vi "Settling Delay Control.vi"(7 "error in":errorcluster, 8 "Settings Cluster":T1={"Supply Voltage [Vdc]"=0.0, "Max Supply Current [Idc]"=0.0, "Settling Delay"=0.0, "Temp Criteria"=0.0, "Voltage Steps [Vrms]"=[], "User Notes"="", "Config Wave File Path"=path "", "Config Voltage [Vrms]"=0.0, "Channel Configuration List"={"Channel Configuration Cluster"={"Input"=enum."---", "Enable"=FALSE, "User Notes"="", "Voltage Range"=15.0, "Current Range"=2.5}, "Channel Configuration Cluster 2"={"Input"=enum."---", "Enable"=FALSE, "User Notes"="", "Voltage Range"=15.0, "Current Range"=2.5}, "Channel Configuration Cluster 3"={"Input"=enum."---", "Enable"=FALSE, "User Notes"="", "Voltage Range"=15.0, "Current Range"=2.5}, "Channel Configuration Cluster 4"={"Input"=enum."---", "Enable"=FALSE, "User Notes"="", "Voltage Range"=15.0, "Current Range"=2.5}, "Channel Configuration Cluster 5"={"Input"=enum."---", "Enable"=FALSE, "User Notes"="", "Voltage Range"=15.0, "Current Range"=2.5}, "Channel Configuration Cluster 6"={"Input"=enum."---", "Enable"=FALSE, "User Notes"="", "Voltage Range"=15.0, "Current Range"=2.5}, "Channel Configuration Cluster 7"={"Input"=enum."---", "Enable"=FALSE, "User Notes"="", "Voltage Range"=15.0, "Current Range"=2.5}, "Channel Configuration Cluster 8"={"Input"=enum."---", "Enable"=FALSE, "User Notes"="", "Voltage Range"=15.0, "Current Range"=2.5}, "Channel Configuration Cluster 9"={"Input"=enum."---", "Enable"=FALSE, "User Notes"="", "Voltage Range"=15.0, "Current Range"=2.5}, "Channel Configuration Cluster 10"={"Input"=enum."---", "Enable"=FALSE, "User Notes"="", "Voltage Range"=15.0, "Current Range"=25.0}, "Channel Configuration Cluster 11"={"Input"=enum."---", "Enable"=FALSE, "User Notes"="", "Voltage Range"=15.0, "Current Range"=25.0}, "Channel Configuration Cluster 12"={"Input"=enum."---", "Enable"=FALSE, "User Notes"="", "Voltage Range"=15.0, "Current Range"=25.0}, "Channel Configuration Cluster 13"={"Input"=enum."---", "Enable"=FALSE, "User Notes"="", "Voltage Range"=15.0, "Current Range"=25.0}, "Channel Configuration Cluster 14"={"Input"=enum."---", "Enable"=FALSE, "User Notes"="", "Voltage Range"=15.0, "Current Range"=25.0}, "Channel Configuration Cluster 15"={"Input"=enum."---", "Enable"=FALSE, "User Notes"="", "Voltage Range"=15.0, "Current Range"=25.0}, "Channel Configuration Cluster 16"={"Input"=enum."---", "Enable"=FALSE, "User Notes"="", "Voltage Range"=15.0, "Current Range"=25.0}, "Channel Configuration Cluster 17"={"Input"=enum."---", "Enable"=FALSE, "User Notes"="", "Voltage Range"=15.0, "Current Range"=25.0}}, "User Gains"={"Gain 1"=0.0, "Gain 2"=0.0, "Gain 3"=0.0, "Gain 4"=0.0, "Gain 5"=0.0, "Gain 6"=0.0}, "Gains"={"Gain 1"=0.0, "Gain 2"=0.0, "Gain 3"=0.0, "Gain 4"=0.0, "Gain 5"=0.0, "Gain 6"=0.0}, "Gain Array"={"Gain 1"=0.0, "Gain 2"=0.0, "Gain 3"=0.0, "Gain 4"=0.0, "Gain 5"=0.0, "Gain 6"=0.0, "Gain 7"=0.0, "Gain 8"=0.0, "Gain 9"=0.0, "Gain 10"=0.0, "Gain 11"=0.0, "Gain 12"=0.0, "Gain 13"=0.0, "Gain 14"=0.0, "Gain 15"=0.0, "Gain 16"=0.0, "Gain 17"=0.0}, "Wave File Path 1"=path "", "Wave File Path 2"=path "", "Wave File Path 3"=path "", "Wave File Path 4"=path "", "Range"=FALSE, "CF"=FALSE} {"Gain Array"."Gain 17" format="%.2f"; "Gain Array"."Gain 16" format="%.2f"; "Gain Array"."Gain 15" format="%.2f"; "Gain Array"."Gain 14" format="%.2f"; "Gain Array"."Gain 13" format="%.2f"; "Gain Array"."Gain 12" format="%.2f"; "Gain Array"."Gain 11" format="%.2f"; "Gain Array"."Gain 10" format="%.2f"; "Gain Array"."Gain 9" format="%.2f"; "Gain Array"."Gain 8" format="%.2f"; "Gain Array"."Gain 7" format="%.2f"; "Gain Array"."Gain 6" format="%.2f"; "Gain Array"."Gain 5" format="%.2f"; "Gain Array"."Gain 4" format="%.2f"; "Gain Array"."Gain 3" format="%.2f"; "Gain Array"."Gain 2" format="%.2f"; "Gain Array"."Gain 1" format="%.2f"; "Gains"."Gain 6" format="%.2f"; "Gains"."Gain 5" format="%.2f"; "Gains"."Gain 4" format="%.2f"; "Gains"."Gain 3" format="%.2f"; "Gains"."Gain 2" format="%.2f"; "Gains"."Gain 1" format="%.2f"; "User Gains"."Gain 6" format="%.2f"; "User Gains"."Gain 5" format="%.2f"; "User Gains"."Gain 4" format="%.2f"; "User Gains"."Gain 3" format="%.2f"; "User Gains"."Gain 2" format="%.2f"; "User Gains"."Gain 1" format="%.2f"; "Channel Configuration List"."Channel Configuration Cluster 17"."Current Range" items=["1 <500m>"=0.5, "2 <1>"=1.0, "5 <2.5>"=2.5, "10 <5>"=5.0, "20 <10>"=10.0, "50 <25>"=25.0]; "Channel Configuration List"."Channel Configuration Cluster 17"."Voltage Range" items=["1.5 <0.75>"=0.75, "3 <1.5>"=1.5, "6 <3>"=3.0, "10 <5>"=5.0, "15 <7.5>"=7.5, "30 <15>"=15.0, "60 <30>"=30.0, "100 <50>"=50.0, "150 <75>"=75.0, "300 <150>"=150.0, "600 <300>"=300.0, "1000 <500>"=500.0]; "Channel Configuration List"."Channel Configuration Cluster 16"."Current Range" items=["1 <500m>"=0.5, "2 <1>"=1.0, "5 <2.5>"=2.5, "10 <5>"=5.0, "20 <10>"=10.0, "50 <25>"=25.0]; "Channel Configuration List"."Channel Configuration Cluster 16"."Voltage Range" items=["1.5 <0.75>"=0.75, "3 <1.5>"=1.5, "6 <3>"=3.0, "10 <5>"=5.0, "15 <7.5>"=7.5, "30 <15>"=15.0, "60 <30>"=30.0, "100 <50>"=50.0, "150 <75>"=75.0, "300 <150>"=150.0, "600 <300>"=300.0, "1000 <500>"=500.0]; "Channel Configuration List"."Channel Configuration Cluster 15"."Current Range" items=["1 <500m>"=0.5, "2 <1>"=1.0, "5 <2.5>"=2.5, "10 <5>"=5.0, "20 <10>"=10.0, "50 <25>"=25.0]; "Channel Configuration List"."Channel Configuration Cluster 15"."Voltage Range" items=["1.5 <0.75>"=0.75, "3 <1.5>"=1.5, "6 <3>"=3.0, "10 <5>"=5.0, "15 <7.5>"=7.5, "30 <15>"=15.0, "60 <30>"=30.0, "100 <50>"=50.0, "150 <75>"=75.0, "300 <150>"=150.0, "600 <300>"=300.0, "1000 <500>"=500.0]; "Channel Configuration List"."Channel Configuration Cluster 14"."Current Range" items=["1 <500m>"=0.5, "2 <1>"=1.0, "5 <2.5>"=2.5, "10 <5>"=5.0, "20 <10>"=10.0, "50 <25>"=25.0]; "Channel Configuration List"."Channel Configuration Cluster 14"."Voltage Range" items=["1.5 <0.75>"=0.75, "3 <1.5>"=1.5, "6 <3>"=3.0, "10 <5>"=5.0, "15 <7.5>"=7.5, "30 <15>"=15.0, "60 <30>"=30.0, "100 <50>"=50.0, "150 <75>"=75.0, "300 <150>"=150.0, "600 <300>"=300.0, "1000 <500>"=500.0]; "Channel Configuration List"."Channel Configuration Cluster 13"."Current Range" items=["1 <500m>"=0.5, "2 <1>"=1.0, "5 <2.5>"=2.5, "10 <5>"=5.0, "20 <10>"=10.0, "50 <25>"=25.0]; "Channel Configuration List"."Channel Configuration Cluster 13"."Voltage Range" items=["1.5 <0.75>"=0.75, "3 <1.5>"=1.5, "6 <3>"=3.0, "10 <5>"=5.0, "15 <7.5>"=7.5, "30 <15>"=15.0, "60 <30>"=30.0, "100 <50>"=50.0, "150 <75>"=75.0, "300 <150>"=150.0, "600 <300>"=300.0, "1000 <500>"=500.0]; "Channel Configuration List"."Channel Configuration Cluster 12"."Current Range" items=["1 <500m>"=0.5, "2 <1>"=1.0, "5 <2.5>"=2.5, "10 <5>"=5.0, "20 <10>"=10.0, "50 <25>"=25.0]; "Channel Configuration List"."Channel Configuration Cluster 12"."Voltage Range" items=["1.5 <0.75>"=0.75, "3 <1.5>"=1.5, "6 <3>"=3.0, "10 <5>"=5.0, "15 <7.5>"=7.5, "30 <15>"=15.0, "60 <30>"=30.0, "100 <50>"=50.0, "150 <75>"=75.0, "300 <150>"=150.0, "600 <300>"=300.0, "1000 <500>"=500.0]; "Channel Configuration List"."Channel Configuration Cluster 11"."Current Range" items=["1 <500m>"=0.5, "2 <1>"=1.0, "5 <2.5>"=2.5, "10 <5>"=5.0, "20 <10>"=10.0, "50 <25>"=25.0]; "Channel Configuration List"."Channel Configuration Cluster 11"."Voltage Range" items=["1.5 <0.75>"=0.75, "3 <1.5>"=1.5, "6 <3>"=3.0, "10 <5>"=5.0, "15 <7.5>"=7.5, "30 <15>"=15.0, "60 <30>"=30.0, "100 <50>"=50.0, "150 <75>"=75.0, "300 <150>"=150.0, "600 <300>"=300.0, "1000 <500>"=500.0]; "Channel Configuration List"."Channel Configuration Cluster 10"."Current Range" items=["1 <500m>"=0.5, "2 <1>"=1.0, "5 <2.5>"=2.5, "10 <5>"=5.0, "20 <10>"=10.0, "50 <25>"=25.0]; "Channel Configuration List"."Channel Configuration Cluster 10"."Voltage Range" items=["1.5 <0.75>"=0.75, "3 <1.5>"=1.5, "6 <3>"=3.0, "10 <5>"=5.0, "15 <7.5>"=7.5, "30 <15>"=15.0, "60 <30>"=30.0, "100 <50>"=50.0, "150 <75>"=75.0, "300 <150>"=150.0, "600 <300>"=300.0, "1000 <500>"=500.0]; "Channel Configuration List"."Channel Configuration Cluster 9"."Voltage Range" items=["1.5 <0.75>"=0.75, "3 <1.5>"=1.5, "6 <3>"=3.0, "10 <5>"=5.0, "15 <7.5>"=7.5, "30 <15>"=15.0, "60 <30>"=30.0, "100 <50>"=50.0, "150 <75>"=75.0, "300 <150>"=150.0, "600 <300>"=300.0, "1000 <500>"=500.0]; "Channel Configuration List"."Channel Configuration Cluster 9"."Current Range" items=["10m <5m>"=0.005, "20m <10m>"=0.01, "50m <25m>"=0.025, "100m <50m>"=0.05, "200m <100m>"=0.1, "500m <250m>"=0.25, "1 <500m>"=0.5, "2 <1>"=1.0, "5 <2.5>"=2.5]; "Channel Configuration List"."Channel Configuration Cluster 8"."Voltage Range" items=["1.5 <0.75>"=0.75, "3 <1.5>"=1.5, "6 <3>"=3.0, "10 <5>"=5.0, "15 <7.5>"=7.5, "30 <15>"=15.0, "60 <30>"=30.0, "100 <50>"=50.0, "150 <75>"=75.0, "300 <150>"=150.0, "600 <300>"=300.0, "1000 <500>"=500.0]; "Channel Configuration List"."Channel Configuration Cluster 8"."Current Range" items=["10m <5m>"=0.005, "20m <10m>"=0.01, "50m <25m>"=0.025, "100m <50m>"=0.05, "200m <100m>"=0.1, "500m <250m>"=0.25, "1 <500m>"=0.5, "2 <1>"=1.0, "5 <2.5>"=2.5]; "Channel Configuration List"."Channel Configuration Cluster 7"."Voltage Range" items=["1.5 <0.75>"=0.75, "3 <1.5>"=1.5, "6 <3>"=3.0, "10 <5>"=5.0, "15 <7.5>"=7.5, "30 <15>"=15.0, "60 <30>"=30.0, "100 <50>"=50.0, "150 <75>"=75.0, "300 <150>"=150.0, "600 <300>"=300.0, "1000 <500>"=500.0]; "Channel Configuration List"."Channel Configuration Cluster 7"."Current Range" items=["10m <5m>"=0.005, "20m <10m>"=0.01, "50m <25m>"=0.025, "100m <50m>"=0.05, "200m <100m>"=0.1, "500m <250m>"=0.25, "1 <500m>"=0.5, "2 <1>"=1.0, "5 <2.5>"=2.5]; "Channel Configuration List"."Channel Configuration Cluster 6"."Voltage Range" items=["1.5 <0.75>"=0.75, "3 <1.5>"=1.5, "6 <3>"=3.0, "10 <5>"=5.0, "15 <7.5>"=7.5, "30 <15>"=15.0, "60 <30>"=30.0, "100 <50>"=50.0, "150 <75>"=75.0, "300 <150>"=150.0, "600 <300>"=300.0, "1000 <500>"=500.0]; "Channel Configuration List"."Channel Configuration Cluster 6"."Current Range" items=["10m <5m>"=0.005, "20m <10m>"=0.01, "50m <25m>"=0.025, "100m <50m>"=0.05, "200m <100m>"=0.1, "500m <250m>"=0.25, "1 <500m>"=0.5, "2 <1>"=1.0, "5 <2.5>"=2.5]; "Channel Configuration List"."Channel Configuration Cluster 5"."Voltage Range" items=["1.5 <0.75>"=0.75, "3 <1.5>"=1.5, "6 <3>"=3.0, "10 <5>"=5.0, "15 <7.5>"=7.5, "30 <15>"=15.0, "60 <30>"=30.0, "100 <50>"=50.0, "150 <75>"=75.0, "300 <150>"=150.0, "600 <300>"=300.0, "1000 <500>"=500.0]; "Channel Configuration List"."Channel Configuration Cluster 5"."Current Range" items=["10m <5m>"=0.005, "20m <10m>"=0.01, "50m <25m>"=0.025, "100m <50m>"=0.05, "200m <100m>"=0.1, "500m <250m>"=0.25, "1 <500m>"=0.5, "2 <1>"=1.0, "5 <2.5>"=2.5]; "Channel Configuration List"."Channel Configuration Cluster 4"."Voltage Range" items=["1.5 <0.75>"=0.75, "3 <1.5>"=1.5, "6 <3>"=3.0, "10 <5>"=5.0, "15 <7.5>"=7.5, "30 <15>"=15.0, "60 <30>"=30.0, "100 <50>"=50.0, "150 <75>"=75.0, "300 <150>"=150.0, "600 <300>"=300.0, "1000 <500>"=500.0]; "Channel Configuration List"."Channel Configuration Cluster 4"."Current Range" items=["10m <5m>"=0.005, "20m <10m>"=0.01, "50m <25m>"=0.025, "100m <50m>"=0.05, "200m <100m>"=0.1, "500m <250m>"=0.25, "1 <500m>"=0.5, "2 <1>"=1.0, "5 <2.5>"=2.5]; "Channel Configuration List"."Channel Configuration Cluster 3"."Voltage Range" items=["1.5 <0.75>"=0.75, "3 <1.5>"=1.5, "6 <3>"=3.0, "10 <5>"=5.0, "15 <7.5>"=7.5, "30 <15>"=15.0, "60 <30>"=30.0, "100 <50>"=50.0, "150 <75>"=75.0, "300 <150>"=150.0, "600 <300>"=300.0, "1000 <500>"=500.0]; "Channel Configuration List"."Channel Configuration Cluster 3"."Current Range" items=["10m <5m>"=0.005, "20m <10m>"=0.01, "50m <25m>"=0.025, "100m <50m>"=0.05, "200m <100m>"=0.1, "500m <250m>"=0.25, "1 <500m>"=0.5, "2 <1>"=1.0, "5 <2.5>"=2.5]; "Channel Configuration List"."Channel Configuration Cluster 2"."Voltage Range" items=["1.5 <0.75>"=0.75, "3 <1.5>"=1.5, "6 <3>"=3.0, "10 <5>"=5.0, "15 <7.5>"=7.5, "30 <15>"=15.0, "60 <30>"=30.0, "100 <50>"=50.0, "150 <75>"=75.0, "300 <150>"=150.0, "600 <300>"=300.0, "1000 <500>"=500.0]; "Channel Configuration List"."Channel Configuration Cluster 2"."Current Range" items=["10m <5m>"=0.005, "20m <10m>"=0.01, "50m <25m>"=0.025, "100m <50m>"=0.05, "200m <100m>"=0.1, "500m <250m>"=0.25, "1 <500m>"=0.5, "2 <1>"=1.0, "5 <2.5>"=2.5]; "Channel Configuration List"."Channel Configuration Cluster"."Voltage Range" items=["1.5 <0.75>"=0.75, "3 <1.5>"=1.5, "6 <3>"=3.0, "10 <5>"=5.0, "15 <7.5>"=7.5, "30 <15>"=15.0, "60 <30>"=30.0, "100 <50>"=50.0, "150 <75>"=75.0, "300 <150>"=150.0, "600 <300>"=300.0, "1000 <500>"=500.0]; "Channel Configuration List"."Channel Configuration Cluster"."Current Range" items=["10m <5m>"=0.005, "20m <10m>"=0.01, "50m <25m>"=0.025, "100m <50m>"=0.05, "200m <100m>"=0.1, "500m <250m>"=0.25, "1 <500m>"=0.5, "2 <1>"=1.0, "5 <2.5>"=2.5]; "Settling Delay" min=0.0 format="%<%H:%M:%S>t"}, 9 "Step Delay Time has Elapsed In":bool, 10 "Reset Delay Clock In":bool, 11 "Step Delay in":dbl) -> (0 "Temperature Data":dbl[](array[numeric]), 1 "Temp Convergence":bool, 2 "Time has Elapsed":bool, 3 "Step Delay out":dbl, 5 "error out":errorcluster)   [LabVIEW 2021]
uses:
  Controls/Settings Control.ctl
  Controls/Channel Configuration List.ctl
  Controls/Channel Configuration Cluster.ctl
  Controls/Channel Configuration Cluster High Current.ctl
  Controls/Gain Averages.ctl
  Controls/Gain Array.ctl
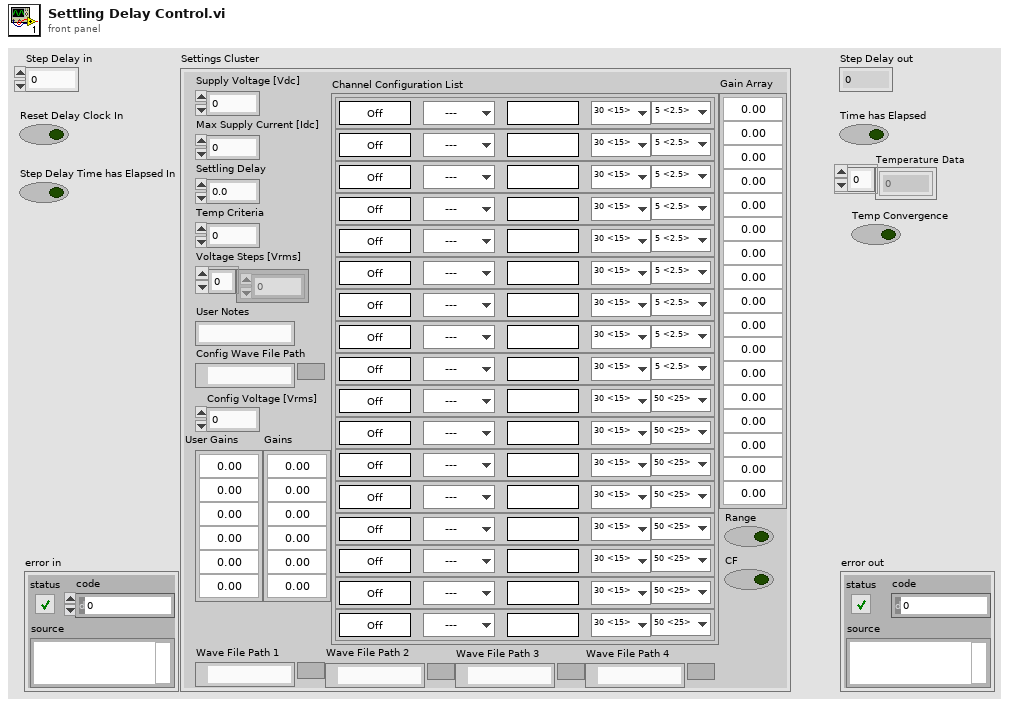
[diagram p1: front panel]
types:
  T1 = typedef "Settings Control.ctl" = cluster{"Supply Voltage [Vdc]":sgl, "Max Supply Current [Idc]":sgl, "Settling Delay":dbl, "Temp Criteria":sgl, "Voltage Steps [Vrms]":sgl[], "User Notes":string, "Config Wave File Path":path, "Config Voltage [Vrms]":sgl, "Channel Configuration List":T2, "User Gains":T5, "Gains":T5, "Gain Array":T6, "Wave File Path 1":path, "Wave File Path 2":path, "Wave File Path 3":path, "Wave File Path 4":path, "Range":bool, "CF":bool}
  T2 = typedef "Channel Configuration List.ctl" = cluster{"Channel Configuration Cluster":T3, "Channel Configuration Cluster 2":T3, "Channel Configuration Cluster 3":T3, "Channel Configuration Cluster 4":T3, "Channel Configuration Cluster 5":T3, "Channel Configuration Cluster 6":T3, "Channel Configuration Cluster 7":T3, "Channel Configuration Cluster 8":T3, "Channel Configuration Cluster 9":T3, "Channel Configuration Cluster 10":T4, "Channel Configuration Cluster 11":T4, "Channel Configuration Cluster 12":T4, "Channel Configuration Cluster 13":T4, "Channel Configuration Cluster 14":T4, "Channel Configuration Cluster 15":T4, "Channel Configuration Cluster 16":T4, "Channel Configuration Cluster 17":T4}
  T3 = typedef "Channel Configuration Cluster.ctl" = cluster{"Input":enum16{"---", "1", "1 AVG", "2", "2 AVG", "3", "3 AVG", "4", "4 AVG"}, "Enable":bool, "User Notes":string, "Voltage Range":dbl, "Current Range":dbl}
  T4 = typedef "Channel Configuration Cluster High Current.ctl" = cluster{"Input":enum16{"---", "1", "1 AVG", "2", "2 AVG", "3", "3 AVG", "4", "4 AVG"}, "Enable":bool, "User Notes":string, "Voltage Range":dbl, "Current Range":dbl}
  T5 = typedef "Gain Averages.ctl" = cluster{"Gain 1":dbl, "Gain 2":dbl, "Gain 3":dbl, "Gain 4":dbl, "Gain 5":dbl, "Gain 6":dbl}
  T6 = typedef "Gain Array.ctl" = cluster{"Gain 1":dbl, "Gain 2":dbl, "Gain 3":dbl, "Gain 4":dbl, "Gain 5":dbl, "Gain 6":dbl, "Gain 7":dbl, "Gain 8":dbl, "Gain 9":dbl, "Gain 10":dbl, "Gain 11":dbl, "Gain 12":dbl, "Gain 13":dbl, "Gain 14":dbl, "Gain 15":dbl, "Gain 16":dbl, "Gain 17":dbl}
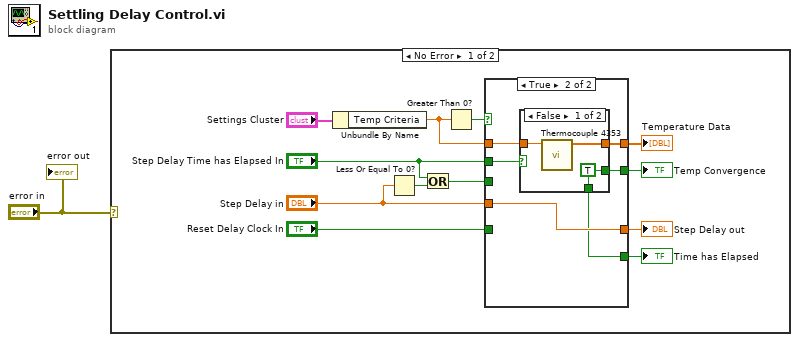
[diagram p0: block diagram]
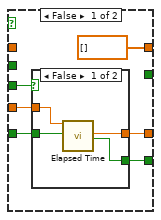
[diagram p2: hidden frame]
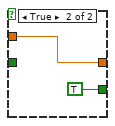
[diagram p3: hidden frame]
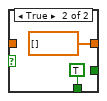
[diagram p4: hidden frame]
diagram:
  n1 = case shown="No Error" "error in" {
    frame No Error {
      n2 = Unbundle By Name("Settings Cluster") -> ("Temp Criteria"=w8:sgl)
      n3 = Less Or Equal To 0?(x="Step Delay in") -> (x <= 0?=w6:bool)
      n4 = Or(x="Step Delay Time has Elapsed In", y=w6) -> (x .or. y?=w4:bool)
      n5 = Greater Than 0?(x=w8) -> (x > 0?=w9:bool)
      n6 = case shown="True" w9 {
        tunnel: [w19 w29] -> w13
        tunnel: "Step Delay Time has Elapsed In" -> [_ w28]
        tunnel: [w18 w31] -> w12
        tunnel: "Reset Delay Clock In" -> [w17 _]
        tunnel: "Step Delay in" -> [w16 w31]
        tunnel: w8 -> [_ w30]
        tunnel: w4 -> [w15 _]
        tunnel: [dbl[] [] ("Temperature Data") w27] -> w3
        tunnel: [_ w26] -> w2
        frame False {
          n7 = case shown="False" w15 {
            tunnel: [w23 TRUE ("Time has Elapsed")] -> w19
            tunnel: w16 -> [w22 w25]
            tunnel: [w21 w25] -> w18
            tunnel: w17 -> [w20 _]
            frame False {
              n8 = call "Elapsed Time"("Time Target (s)"=w22, "Reset"=w20) -> ("Elapsed Time (s)"=w21:dbl, "Time has Elapsed"=w23:bool)  [unwired: 10 in, 6 out]
            }
            frame True {
            }
          }
        }
        frame True {
          n9 = case shown="False" w28 {
            tunnel: w30 -> [w34 _]
            tunnel: [w32 TRUE ("Time has Elapsed")] -> w29
            tunnel: [w33 dbl[] [] ("Temperature Data")] -> w27
            tunnel: [w32 _] -> w26
            frame False {
              w32 = TRUE ("Time has Elapsed")
              n10 = call "Thermocouple 4353 .vi"("Temp Convergence Criteria [deg C]"=w34) -> ("Temperature Data"=w33:dbl[])  [unwired: 10 in]
            }
            frame True {
            }
          }
        }
      }
      "Time has Elapsed" <- w13
      "Step Delay out" <- w12
      "Temperature Data" <- w3
      "Temp Convergence" <- w2
    }
    frame Error {
    }
  }
  "error out" <- "error in"
